vi "Event Sequencer Next.vi"(1 "Enum in":T1) -> (0 "Enum out":T1)   [LabVIEW 2016]
uses:
  type-defs/TD_Event Sequencer.ctl
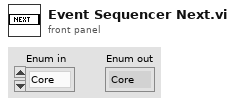
[diagram p1: front panel]
types:
  T1 = typedef "TD_Event Sequencer.ctl" = enum16{"Core", "Plugins"}
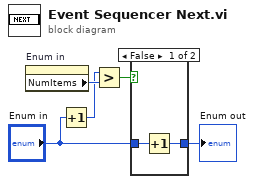
[diagram p0: block diagram]
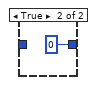
[diagram p2: hidden frame]
diagram:
  n1 = property on="Enum in" class="Enum (strict)"() -> ("NumItems"=w3:u32)  [unwired: 2 in, 2 out]
  n2 = Increment(x="Enum in") -> (x+1=w1:T1)
  n3 = Greater?(x=w1, y=w3) -> (0:w2:bool)
  n4 = case shown="False" w2 {
    tunnel: [w7 0] -> w5
    tunnel: "Enum in" -> [w6 _]
    frame False {
      n5 = Increment(x=w6) -> (x+1=w7:T1)
    }
    frame True {
    }
  }
  "Enum out" <- w5
